vi "Write FPGA Ref.vi"(8 "error in (no error)":errorcluster, 10 "FPGA Ref":T1, 11 "tCRD in":refnum<class "tCRD.lvclass">) -> (0 "error out":errorcluster, 3 "tCRD out":refnum<class "tCRD.lvclass">)   [LabVIEW 2015, in "tCRD.lvclass"]
uses:
  tCRD.lvclass
  tFPGA Ref.ctl
  tCRD.lvclass/tCRD.ctl
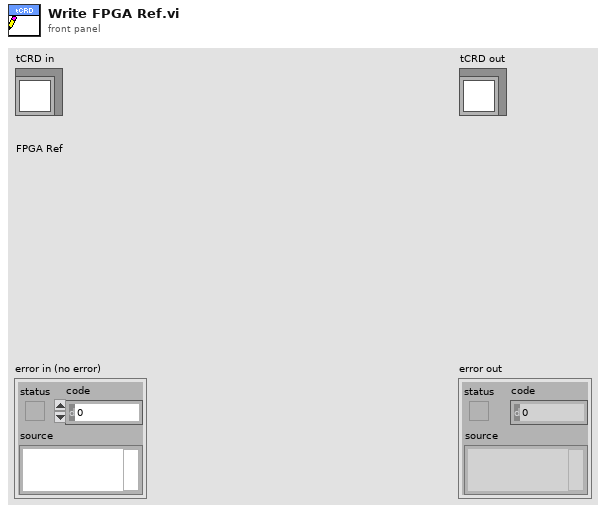
[diagram p1: front panel]
types:
  T1 = typedef "tCRD.lvclass/tFPGA Ref.ctl" = refnum<k20>
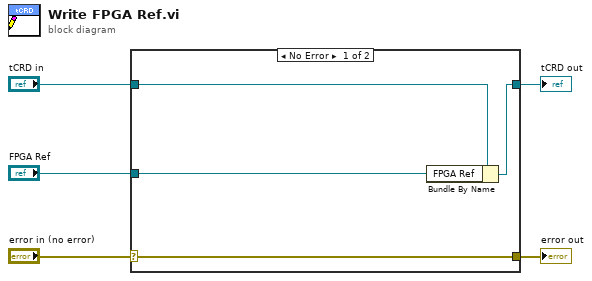
[diagram p0: block diagram]
diagram:
  n1 = case shown="No Error" "error in (no error)" {
    selector: "error in (no error)" -> [w9 w10]
    tunnel: [w9 w10] -> w4
    tunnel: [w7 w11] -> w2
    tunnel: "tCRD in" -> [w8 w11]
    tunnel: "FPGA Ref" -> [w6 _]
    frame No Error {
      n2 = Bundle By Name(cluster=w8, "FPGA Ref"=w6) -> (w7:refnum<class "tCRD.lvclass">)
    }
    frame Error {
    }
  }
  "error out" <- w4
  "tCRD out" <- w2
